vi "TOI Fetch Data (ALL) - TOI.vi"(8 "error in (no error)":errorcluster, 10 "Current Settings":T2, 11 "Refnum in":refnum<k21>) -> (0 "error out":errorcluster, 1 "IM Spectrum":cluster{"x0":dbl, "dx":dbl, "y":sgl[]}[](graph), 2 "Data Cluster":T1, 3 "Refnum out":refnum<k21>)   [LabVIEW 2023]
uses:
  Controls/Data Cluster - Settings - TOI.ctl
  Controls/Data Cluster - TOI.ctl
  <vilib>/RFmx/SpecAn/mx/RFmxSpecAn.llb/RFmxSpecAn IM Fetch Fundamental Measurement.vi
  <vilib>/RFmx/SpecAn/mx/RFmxSpecAn.llb/RFmxSpecAn IM Fetch Intermod Measurement.vi
  <vilib>/RFmx/SpecAn/mx/RFmxSpecAn.llb/RFmxSpecAn IM Fetch Intercept Power.vi
  <vilib>/RFmx/SpecAn/mx/RFmxSpecAn.llb/RFmxSpecAn IM Fetch Spectrum.vi
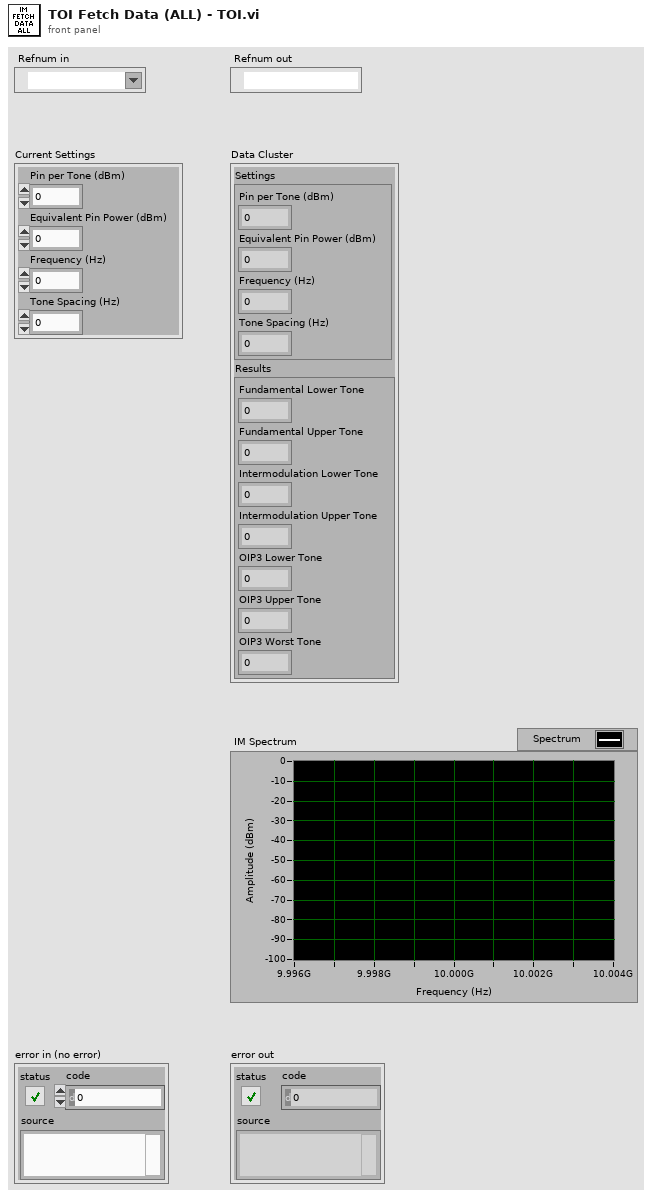
[diagram p1: front panel]
types:
  T1 = typedef "Data Cluster - TOI.ctl" = cluster{"Settings":T2, "Results":cluster{"Fundamental Lower Tone":dbl, "Fundamental Upper Tone":dbl, "Intermodulation Lower Tone":dbl, "Intermodulation Upper Tone":dbl, "OIP3 Lower Tone":dbl, "OIP3 Upper Tone":dbl, "OIP3 Worst Tone":dbl}}
  T2 = typedef "Data Cluster - Settings - TOI.ctl" = cluster{"Pin per Tone (dBm)":dbl, "Equivalent Pin Power (dBm)":dbl, "Frequency (Hz)":dbl, "Tone Spacing (Hz)":dbl}
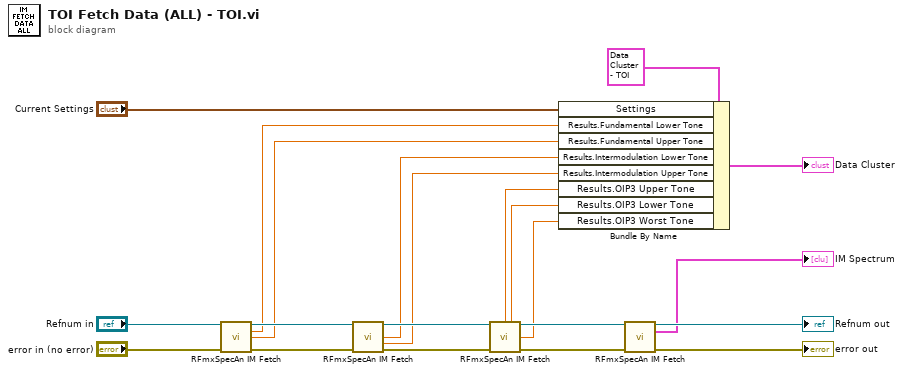
[diagram p0: block diagram]
diagram:
  n1 = call-poly <vilib>:"RFmxSpecAn IM Fetch.vi"("Instrument Handle In"="Refnum in", "error in (no error)"="error in (no error)") -> ("Instrument Handle Out"=w13:refnum<k21>, "Lower Tone Power (dBm)"=w9:dbl, "Upper Tone Power (dBm)"=w10:dbl, "error out"=w14:errorcluster)  [unwired: 10 in]
  n2 = call-poly <vilib>:"RFmxSpecAn IM Fetch.vi"("Instrument Handle In"=w13, "error in (no error)"=w14) -> ("Instrument Handle Out"=w16:refnum<k21>, "Lower Intermod Absolute Power (dBm)"=w7:dbl, "Upper Intermod Absolute Power (dBm)"=w8:dbl, "error out"=w15:errorcluster)  [unwired: 9 in, 1 out]
  n3 = call-poly <vilib>:"RFmxSpecAn IM Fetch.vi"("Instrument Handle In"=w16, "error in (no error)"=w15) -> ("Upper Output Intercept Power (dBm)"=w2:dbl, "Lower Output Intercept Power (dBm)"=w1:dbl, "Instrument Handle Out"=w17:refnum<k21>, "Worst Case Output Intercept Power (dBm)"=w11:dbl, "error out"=w18:errorcluster)  [unwired: 8 in, 1 out]
  n4 = Bundle By Name(cluster=T1 {"Settings"={"Pin per Tone (dBm)"=-20.0, "Equivalent Pin Power (dBm)"=-20.0, "Frequency (Hz)"=10000000000.0, "Tone Spacing (Hz)"=1000000.0}, "Results"={"Fundamental Lower Tone"=0.0, "Fundamental Upper Tone"=0.0, "Intermodulation Lower Tone"=0.0, "Intermodulation Upper Tone"=0.0, "OIP3 Lower Tone"=0.0, "OIP3 Upper Tone"=0.0, "OIP3 Worst Tone"=0.0}} ("Cluster"), "Settings"="Current Settings", "Results.Fundamental Lower Tone"=w9, "Results.Fundamental Upper Tone"=w10, "Results.Intermodulation Lower Tone"=w7, "Results.Intermodulation Upper Tone"=w8, "Results.OIP3 Upper Tone"=w2, "Results.OIP3 Lower Tone"=w1, "Results.OIP3 Worst Tone"=w11) -> (→"Data Cluster":T1)
  n5 = call-poly <vilib>:"RFmxSpecAn IM Fetch.vi"("Instrument Handle In"=w17, "error in (no error)"=w18) -> ("Instrument Handle Out"=→"Refnum out":refnum<k21>, "Spectrums (dBm)"=→"IM Spectrum":cluster{"x0":dbl, "dx":dbl, "y":sgl[]}[], "error out"=→"error out":errorcluster)  [unwired: 11 in]
